vi "Pack Publish Request.vi"(6 "Publication Time (Use Current Time)":timestamp, 7 "Publisher ID":string, 8 "error in (no error)":errorcluster, 9 "Value":variant, 10 "Datum Name":string, 11 "PublishRequest In":refnum<class "PublishRequest.lvclass">) -> (0 "error out":errorcluster, 3 "PublishRequest Out":refnum<class "PublishRequest.lvclass">)   [LabVIEW 2017, in "IMediator.lvlib" / "PublishRequest.lvclass"]
uses:
  <vilib>/gpm_packages/@cs/mva-core/Source/IMediator/PublishRequest/PublishRequest.lvclass
  <vilib>/gpm_packages/@cs/mva-core/Source/IMediator/PublishRequest/PublishRequest.lvclass/PublishRequest.ctl
  <vilib>/Utility/error.llb/Error Cluster From Error Code.vi
  <vilib>/ErrorRing/Error Ring.xnode
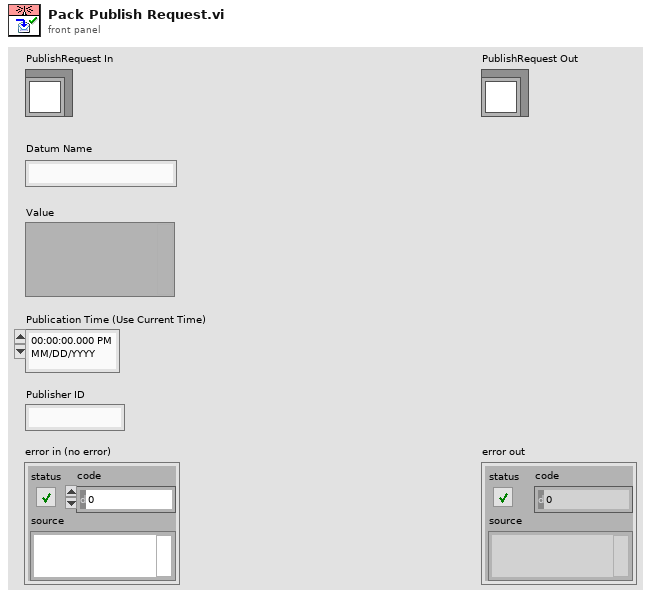
[diagram p1: front panel]
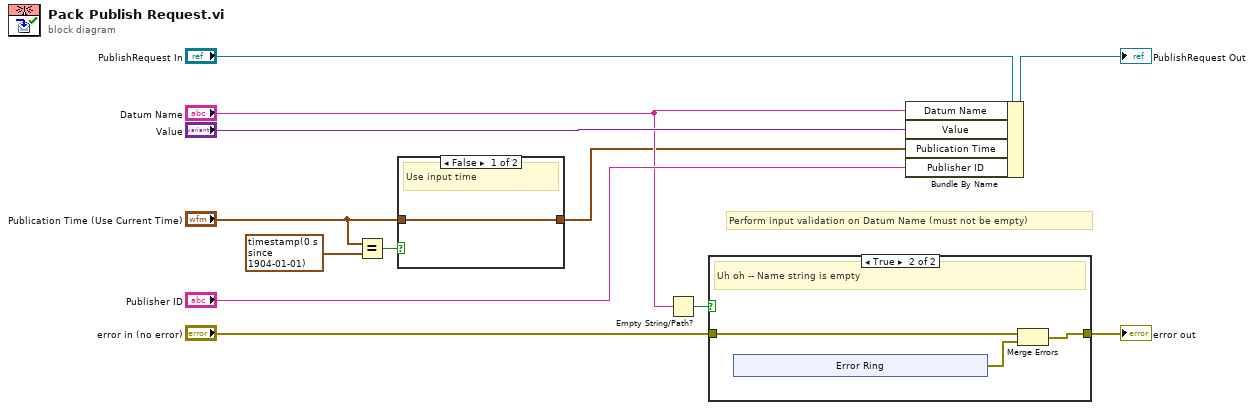
[diagram p0: block diagram]
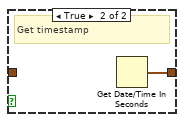
[diagram p3: hidden frame]
diagram:
  # "Perform input validation on Datum Name (must not be empty)"
  n1 = Equal?(x="Publication Time (Use Current Time)", y=timestamp(0 s since 1904-01-01)) -> (x = y?=w3:bool)
  n2 = case shown="False" w3 {
    tunnel: "Publication Time (Use Current Time)" -> [w13 _]
    tunnel: [w13 w14] -> w4
    frame False {
      # "Use input time"
    }
    frame True {
      # "Get timestamp"
      n3 = Get Date/Time In Seconds() -> (seconds since 1Jan1904=w14:timestamp)
    }
  }
  n4 = Empty String/Path?(string/path="Datum Name") -> (empty?=w1:bool)
  n5 = case shown="True" w1 {
    tunnel: "error in (no error)" -> [w15 w18]
    tunnel: [w15 w17] -> w5
    frame False {
      # "No problem!"
    }
    frame True {
      # "Uh oh -- Name string is empty"
      n6 = xnode "Error Ring"() -> ("error out"=w16:errorcluster)
      n7 = Merge Errors(w18, w16) -> (w17:errorcluster)
    }
  }
  "error out" <- w5
  n8 = Bundle By Name(cluster="PublishRequest In", "Datum Name"="Datum Name", "Value"="Value", "Publication Time"=w4, "Publisher ID"="Publisher ID") -> (→"PublishRequest Out":refnum<class "PublishRequest.lvclass">)
